vi "Tank Drive.vi"(1 "Joy y1":dbl, 4 "Joy y2":dbl) -> (12 "rot FL":dbl, 13 "Drive FL":dbl, 14 "rot FR":dbl, 15 "rot BL":dbl, 16 "rot BR":dbl, 17 "Drive FR":dbl, 18 "Drive BL":dbl, 19 "Drive BR":dbl)   [LabVIEW 2014]
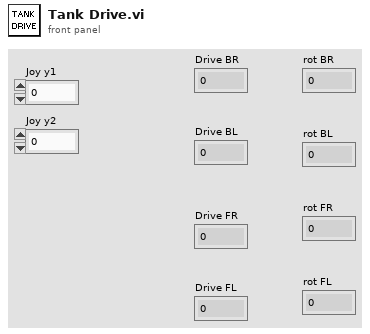
[diagram p1: front panel]
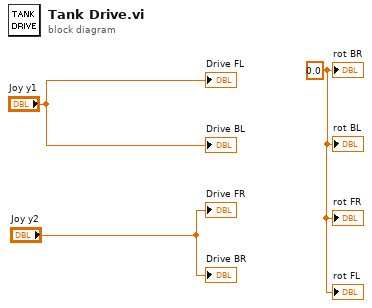
[diagram p0: block diagram]
diagram:
  w3 = 0.0 ("rot BR")
  "rot BR" <- w3
  "rot BL" <- w3
  "rot FR" <- w3
  "rot FL" <- w3
  "Drive BR" <- "Joy y2"
  "Drive BL" <- "Joy y1"
  "Drive FR" <- "Joy y2"
  "Drive FL" <- "Joy y1"
